vi "circle generator.vi"(6 "end":dbl=360.0, 7 "start":dbl format="%#_13g", 9 "r":dbl=1.0, 10 "yc":dbl format="%#_13g", 11 "xc":dbl) -> (0 "y":dbl[](array[numeric]), 1 "x":dbl[](array[numeric]), 3 "graph":cluster{dbl[], dbl[]}(graph))   [LabVIEW 2014]
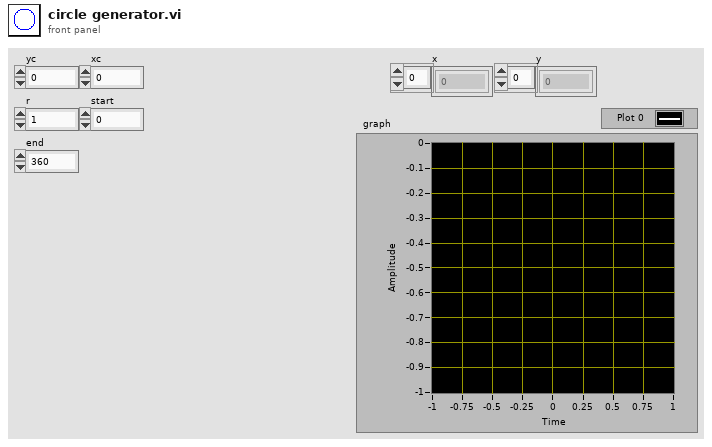
[diagram p1: front panel]
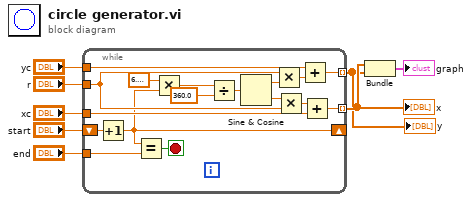
[diagram p0: block diagram]
diagram:
  n1 = while {
    tunnel: "r" -> [w14]
    tunnel: "xc" -> [w15]
    tunnel: "yc" -> [w23]
    tunnel: [w21] -> w8 mode=indexing
    tunnel: [w20] -> w7 mode=indexing
    shift-right: [w12] -> _
    shift-left: "start" -> [w11]
    tunnel: "end" -> [w10]
    stop <- w19 stop-if-true
    n2 = Increment(x=w11) -> (x+1=w12:dbl)
    n3 = Equal?(x=w12, y=w10) -> (x = y?=w19:bool)
    n4 = Multiply(x=6.283185307179586, y=w12) -> (x*y=w24:dbl)
    n5 = Divide(x=w24, y=360.0) -> (x/y=w18:dbl)
    n6 = Sine & Cosine(0:w18) -> (1:w17:dbl, 2:w13:dbl)
    n7 = Multiply(x=w14, y=w17) -> (x*y=w22:dbl)
    n8 = Multiply(x=w13, y=w14) -> (x*y=w16:dbl)
    n9 = Add(x=w23, y=w22) -> (x+y=w20:dbl)
    n10 = Add(x=w16, y=w15) -> (x+y=w21:dbl)
  }
  "x" <- w8
  "y" <- w7
  n11 = Bundle(w8, w7) -> (→"graph":cluster{dbl[], dbl[]})  [unwired: 1 in]
